vi "GetMarkerMode.vi"(3 "error in (no error)":errorcluster, 4 "Marker (0: Marker 1)":u16(ring) items=["Marker 1", "Marker 2", "Marker 3", "Marker 4"], 5 "VISA resource name":refnum<visa-resource-name>) -> (0 "error out":errorcluster, 1 "Marker Mode":u8(ring) items=["Fixed Low", "Fixed High", "Automatic", "Replicate Digital 0"], 2 "VISA resource name out":refnum<visa-resource-name>)   [LabVIEW 2020, in "Active Technologies AWG3000.lvlib"]
uses:
  Active Technologies AWG3000.lvlib
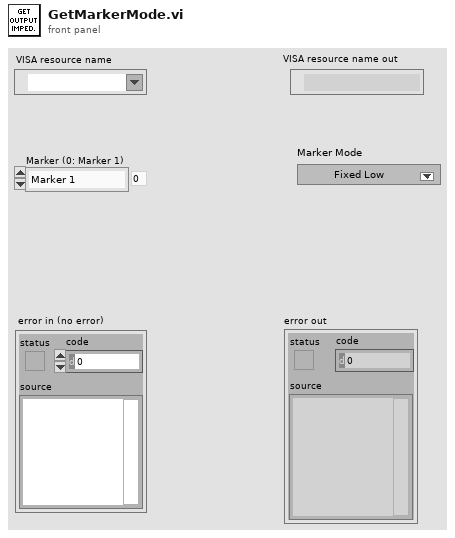
[diagram p1: front panel]
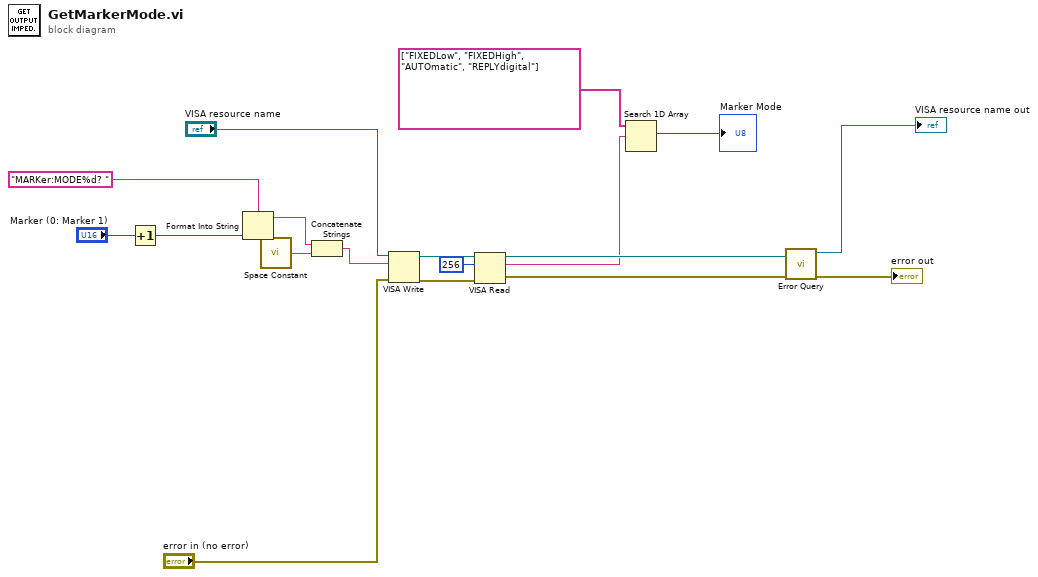
[diagram p0: block diagram]
diagram:
  n1 = Increment(x="Marker (0: Marker 1)") -> (x+1=w14:u16)
  n2 = Format Into String(format string="MARKer:MODE%d? " ("write buffer"), w14) -> (resulting string=w13:string)  [unwired: 2 in, 1 out]
  n3 = call <vilib>:"Space Constant.vi"() -> ("String"=w4:string)
  n4 = Concatenate Strings(w13, w4) -> (w12:string)
  n5 = VISA Write(VISA resource name="VISA resource name", write buffer=w12, error in (no error)="error in (no error)") -> (VISA resource name out=w11:refnum<visa-resource-name>, error out=w10:errorcluster)  [unwired: 1 out]
  n6 = VISA Read(VISA resource name=w11, byte count=u32 256, error in (no error)=w10) -> (VISA resource name out=w8:refnum<visa-resource-name>, read buffer=w2:string, error out=w7:errorcluster)  [unwired: 1 out]
  n7 = Search 1D Array(1D array=string[] ["FIXEDLow", "FIXEDHigh", "AUTOmatic", "REPLYdigital"], element=w2) -> (index of element=→"Marker Mode":i32)  [unwired: 1 in]
  n8 = call "Error Query.vi"("error in (no error)"=w7, "VISA resource name"=w8) -> ("error out"=→"error out":errorcluster, "VISA resource name out"=→"VISA resource name out":refnum<visa-resource-name>)  [unwired: 6 in, 2 out]
